vi "SimpleLiveAppPostProcessing.vi"() -> ()   [LabVIEW 2018]
uses:
  D:/SVN/PM/sdk/AppSamples/LabVIEWSamples/trunk/Release/2018/Dependencies/PVCamNET.dll
  Dependencies/PVCamNET.dll
panel:
  in  "Value":dbl
  in  "Post Processing":string(combo)
  in  "Exposure Time":dbl
  in  "Live":bool
  in  "Camera Status":bool
  in  "Uninit":bool
  in  "Live stop":bool
  in  "Live start":bool
  in  "Init":bool
  # "SimpleLiveAppPostProcessing.vi\n\nDescription:\nThis sample code lets the user use post processing\nfeature in an event driven structure.\n\nSteps to run:\n1. Click \"Run\"\n2. Click \"Open\"\n3. Enter Exposure Time\n4. Choose Post Processing feature\n5. Update Value\n6. Click \"Live start\"\n7. Click \"Live stop\"\n8. Click \"Close\""
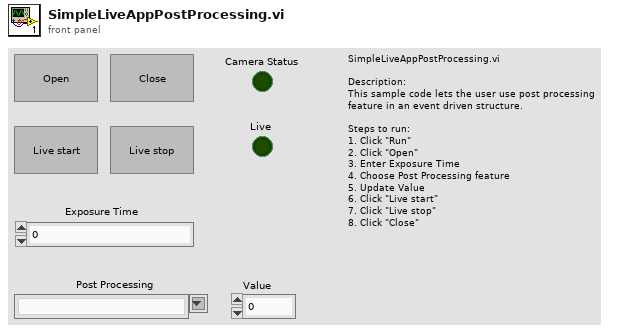
[diagram p1: front panel]
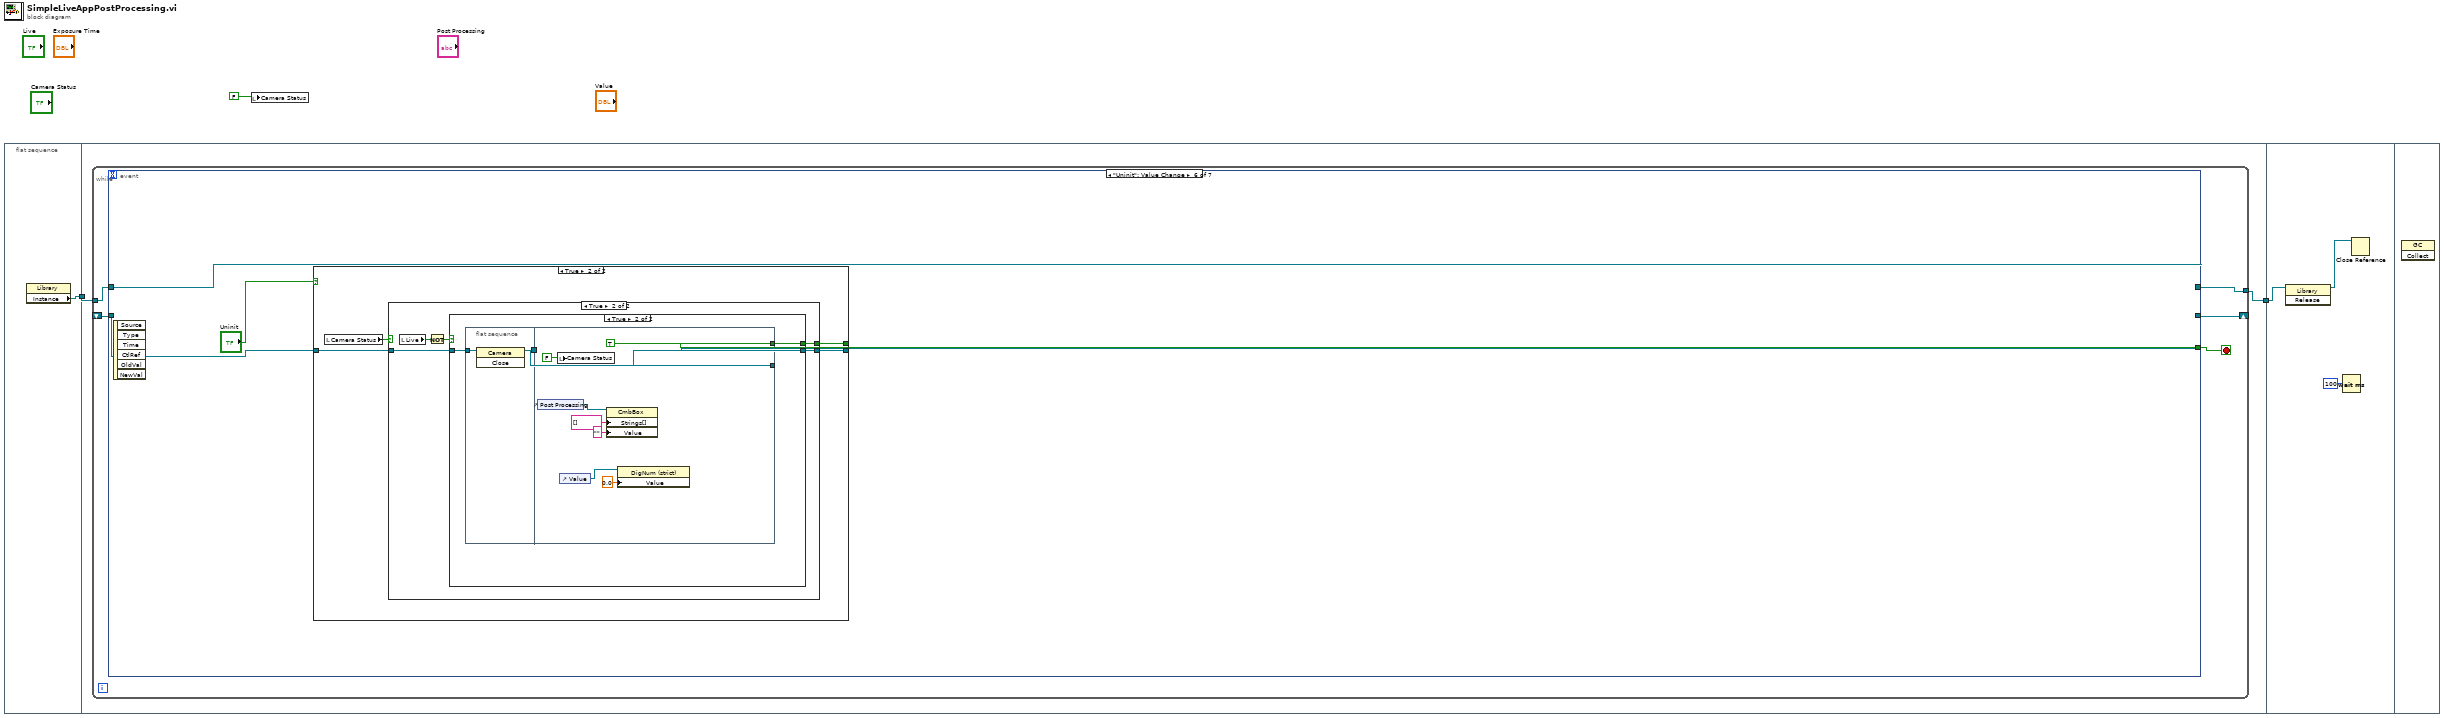
[diagram p0: block diagram]
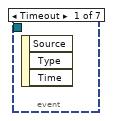
[diagram p2: hidden frame]
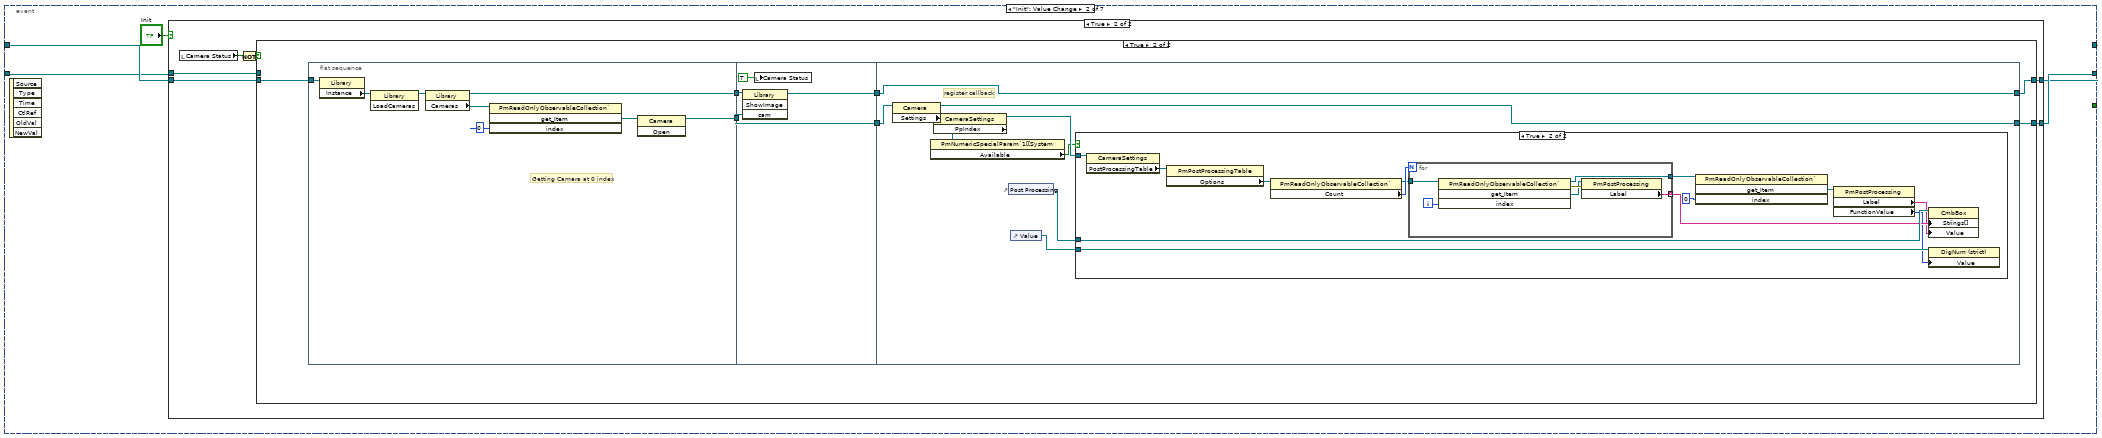
[diagram p3: hidden frame]
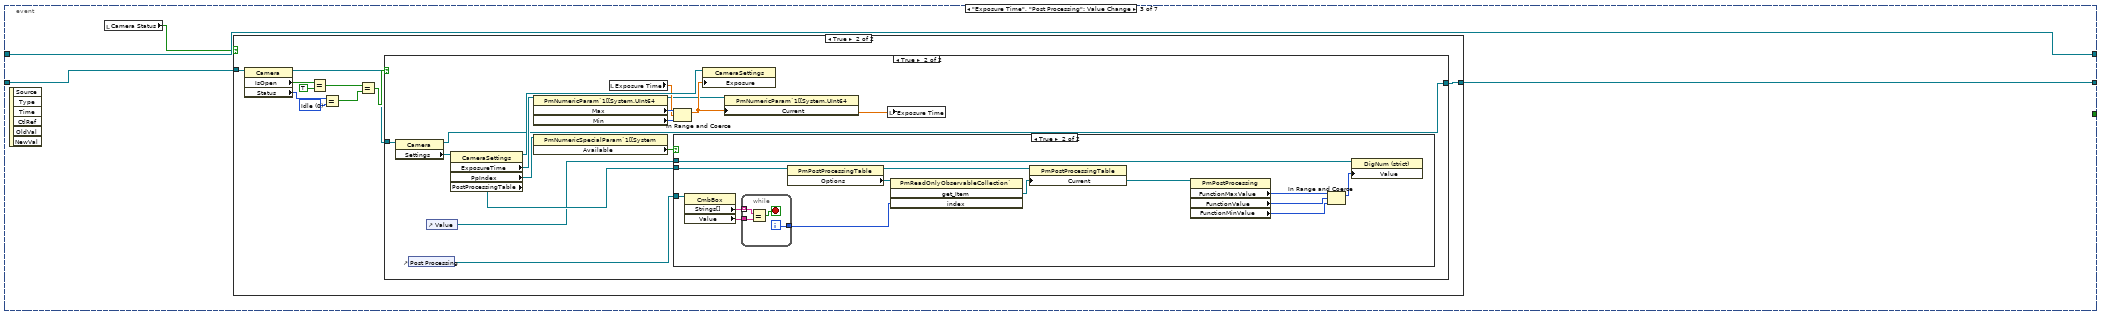
[diagram p7: hidden frame]
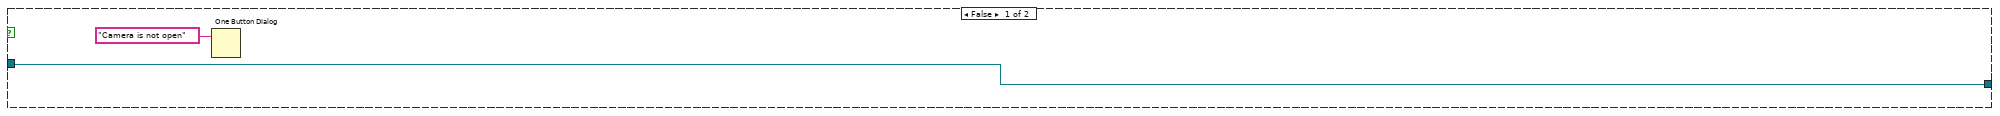
[diagram p8: hidden frame]
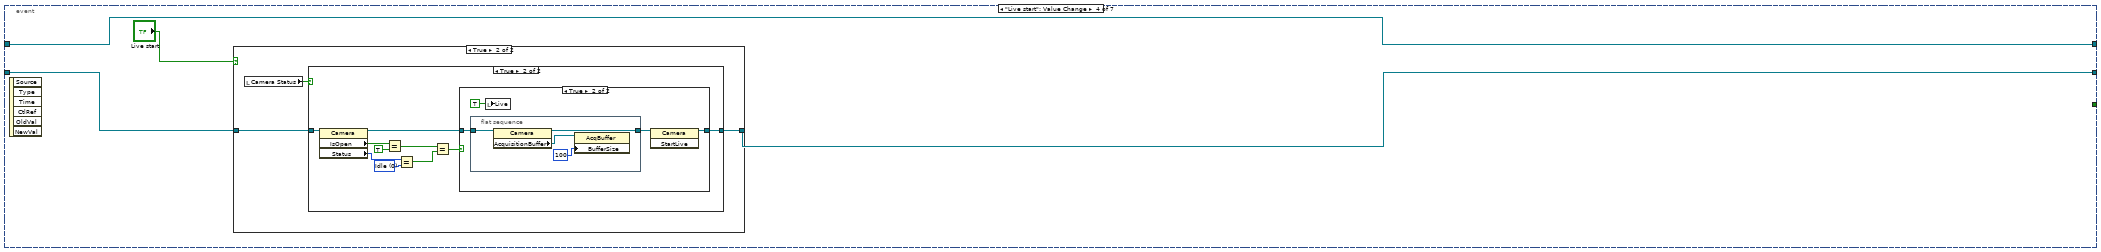
[diagram p11: hidden frame]
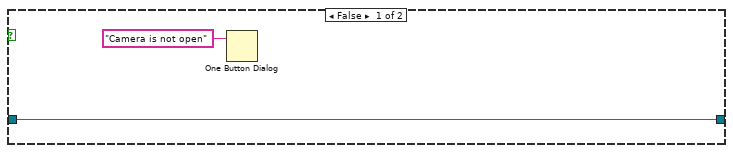
[diagram p13: hidden frame]
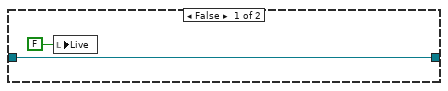
[diagram p14: hidden frame]
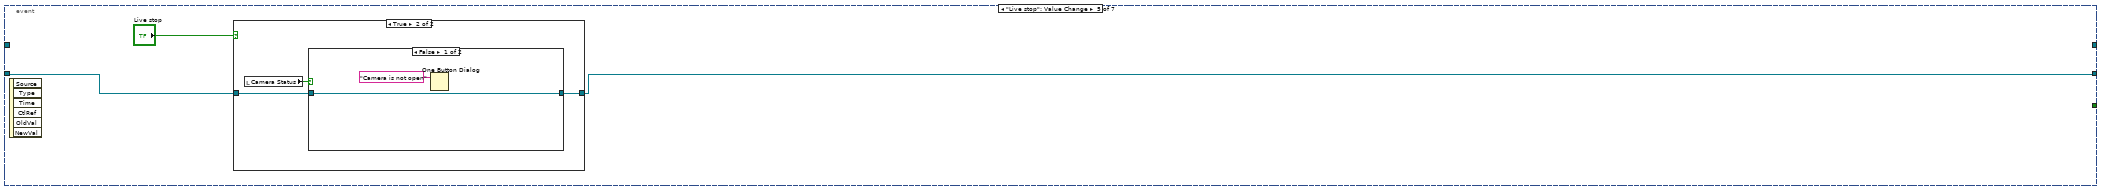
[diagram p15: hidden frame]
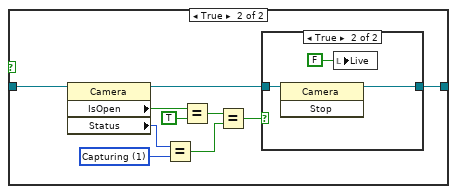
[diagram p17: hidden frame]
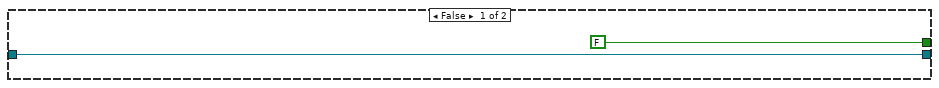
[diagram p19: hidden frame]
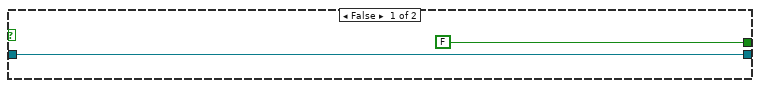
[diagram p20: hidden frame]
diagram:
  n1 = flat-sequence {
    tunnel: [w4] -> w3
    tunnel: w3 -> [w6]
    tunnel: [w5] -> w2
    tunnel: w2 -> [w243]
    frame #0 {
      n2 = property class="Library"() -> ("Instance"=w4:refnum<k24>)  [unwired: 2 in, 2 out]
    }
    frame #1 {
      n3 = while {
        tunnel: w6 -> [w11]
        shift-right: [w10] -> _
        shift-left: _ -> [w8]
        tunnel: [w9] -> w5
        stop <- w7 stop-if-true
        n4 = event shown="[5] \"Uninit\": Value Change" {
          selector: _ -> [_ _ _ _ _ _ _]
          dyn-events: _ -> [_ _ _ _ _ _ _]
          timeout: _ -> [_ _ _ _ _ _ _]
          tunnel: w11 -> [_ w16 w75 w123 _ w178 _]
          tunnel: [_ w15 w76 w124 w153 w179 w210] -> w10
          tunnel: [_ w14 w75 w123 _ w178 _] -> w9
          tunnel: w8 -> [_ w13 w77 w125 w154 w180 w212]
          tunnel: [_ _ _ _ _ w177 _] -> w7
          event Timeout {
            n5 = event-data() -> ()  [unwired: 1 in, 3 out]
          }
          event "Init": Value Change {
            n6 = event-data() -> ()  [unwired: 1 in, 6 out]
            n7 = case shown="True" "Init" {
              tunnel: w16 -> [w18 w24]
              tunnel: [w17 w23] -> w15
              tunnel: [w18 w22] -> w14
              tunnel: w13 -> [w17 w19]
              frame False {
              }
              frame True {
                n8 = local read "Camera Status"() -> (w21:bool)
                n9 = Not(x=w21) -> (.not. x?=w20:bool)
                n10 = case shown="True" w20 {
                  tunnel: w24 -> [w25 w31]
                  tunnel: [w26 w30] -> w23
                  tunnel: [w25 w29] -> w22
                  tunnel: w19 -> [w26 _]
                  frame False {
                  }
                  frame True {
                    n11 = flat-sequence {
                      tunnel: w31 -> [w37]
                      tunnel: [w38] -> w33
                      tunnel: [w34] -> w32
                      tunnel: w33 -> [w44]
                      tunnel: w32 -> [w45]
                      tunnel: [w45] -> w28
                      tunnel: [w43] -> w27
                      tunnel: [w54] -> w29
                      tunnel: [w46] -> w30
                      tunnel: w28 -> [w47]
                      tunnel: w27 -> [w54]
                      frame #0 {
                        # "Getting Camera at 0 index"
                        n12 = property class="Library"(reference=w37) -> ("Instance"=w36:refnum<k24>)  [unwired: 1 in, 2 out]
                        n13 = invoke class="Library" method="LoadCameras"(reference=w36) -> (reference out=w35:refnum<k24>)  [unwired: 2 in, 2 out]
                        n14 = property class="Library"(reference=w35) -> (reference out=w38:refnum<k24>, "Cameras"=w41:refnum<k24>)  [unwired: 1 in, 1 out]
                        n15 = invoke class="PmReadOnlyObservableCollection`" method="get_Item"(reference=w41, "index"=0) -> ("get_Item"=w39:refnum<k24>)  [unwired: 2 in, 3 out]
                        n16 = invoke class="Camera" method="Open"(reference=w39) -> (reference out=w34:refnum<k24>)  [unwired: 2 in, 2 out]
                      }
                      frame #1 {
                        n17 = invoke class="Library" method="ShowImage"(reference=w44, "cam"=w45) -> (reference out=w43:refnum<k24>)  [unwired: 2 in, 3 out]
                        n18 = local write "Camera Status"(TRUE ("Camera Status")) -> ()
                      }
                      frame #2 {
                        # "register callback"
                        n19 = property class="Camera"(reference=w47) -> (reference out=w46:refnum<k24>, "Settings"=w50:refnum<k24>)  [unwired: 1 in, 1 out]
                        n20 = property class="CameraSettings"(reference=w50) -> (reference out=w51:refnum<k24>, "PpIndex"=w49:refnum<k24>)  [unwired: 1 in, 1 out]
                        n21 = property class="PmNumericSpecialParam`1[[System"(reference=w49) -> ("Available"=w48:bool)  [unwired: 1 in, 2 out]
                        n22 = control-ref of="Post Processing"() -> (w52:refnum<vi>)
                        n23 = control-ref of="Value"() -> (w53:refnum<vi>)
                        n24 = case shown="True" w48 {
                          tunnel: w51 -> [_ w67]
                          tunnel: w52 -> [_ w59]
                          tunnel: w53 -> [_ w56]
                          frame False {
                          }
                          frame True {
                            n25 = property class="CameraSettings"(reference=w67) -> ("PostProcessingTable"=w66:refnum<k24>)  [unwired: 1 in, 2 out]
                            n26 = property class="PmPostProcessingTable"(reference=w66) -> ("Options"=w65:refnum<k24>)  [unwired: 1 in, 2 out]
                            n27 = property class="PmReadOnlyObservableCollection`"(reference=w65) -> (reference out=w63:refnum<k24>, "Count"=w64:i32)  [unwired: 1 in, 1 out]
                            n28 = for {
                              N: w64 -> [_]
                              tunnel: w63 -> [w73]
                              tunnel: [w69] -> w58 mode=indexing
                              tunnel: [w68] -> w62
                              i -> [w72]
                              n29 = invoke class="PmReadOnlyObservableCollection`" method="get_Item"(reference=w73, "index"=w72) -> (reference out=w68:refnum<k24>, error out=w71:errorcluster, "get_Item"=w70:refnum<k24>)  [unwired: 2 in, 1 out]
                              n30 = property class="PmPostProcessing"(reference=w70, error in=w71) -> ("Label"=w69:string)  [unwired: 2 out]
                            }
                            n31 = invoke class="PmReadOnlyObservableCollection`" method="get_Item"(reference=w62, "index"=0) -> ("get_Item"=w60:refnum<k24>)  [unwired: 2 in, 3 out]
                            n32 = property class="PmPostProcessing"(reference=w60) -> ("Label"=w57:string, "FunctionValue"=w55:i32)  [unwired: 1 in, 2 out]
                            n33 = property class="CmbBox"(reference=w59, "Strings[]"=w58, "Value"=w57) -> ()  [unwired: 1 in, 2 out]
                            n34 = property class="DigNum (strict)"(reference=w56, "Value"=w55) -> ()  [unwired: 1 in, 2 out]
                          }
                        }
                      }
                    }
                  }
                }
              }
            }
          }
          event "Exposure Time", "Post Processing": Value Change {
            n35 = event-data() -> ()  [unwired: 1 in, 6 out]
            n36 = local read "Camera Status"() -> (w74:bool)
            n37 = case shown="True" w74 {
              tunnel: w77 -> [w79 w83]
              tunnel: [w79 w80] -> w76
              frame False {
                n38 = One Button Dialog(message="Camera is not open") -> ()  [unwired: 1 in, 1 out]
              }
              frame True {
                w88 = 0 items=["Idle", "Capturing"] ("Status")
                n39 = property class="Camera"(reference=w83) -> (reference out=w81:refnum<k24>, "IsOpen"=w87:bool, "Status"=w89:i32)  [unwired: 1 in, 1 out]
                n40 = Equal?(x=w87, y=TRUE) -> (x = y?=w85:bool)
                n41 = Equal?(x=w89, y=w88) -> (x = y?=w84:bool)
                n42 = Equal?(x=w85, y=w84) -> (x = y?=w82:bool)
                n43 = case shown="True" w82 {
                  tunnel: w81 -> [w90 w105]
                  tunnel: [w90 w98] -> w80
                  frame False {
                  }
                  frame True {
                    n44 = property class="Camera"(reference=w105) -> (reference out=w98:refnum<k24>, "Settings"=w104:refnum<k24>)  [unwired: 1 in, 1 out]
                    n45 = control-ref of="Post Processing"() -> (w95:refnum<vi>)
                    n46 = control-ref of="Value"() -> (w93:refnum<vi>)
                    n47 = property class="CameraSettings"(reference=w104) -> (reference out=w100:refnum<k24>, "ExposureTime"=w101:refnum<k24>, "PpIndex"=w97:refnum<k24>, "PostProcessingTable"=w94:refnum<k24>)  [unwired: 1 in, 1 out]
                    n48 = property class="PmNumericParam`1[[System.UInt64"(reference=w101) -> (reference out=w91:refnum<k24>, "Max"=w103:u64, "Min"=w102:u64)  [unwired: 1 in, 1 out]
                    n49 = property class="PmNumericSpecialParam`1[[System"(reference=w97) -> ("Available"=w96:bool)  [unwired: 1 in, 2 out]
                    n50 = local read "Exposure Time"() -> (w99:dbl)
                    n51 = In Range and Coerce(upper limit=w103, x=w99, lower limit=w102) -> (coerced(x)=w92:dbl)  [unwired: 1 out]
                    n52 = case shown="True" w96 {
                      tunnel: w94 -> [_ w108]
                      tunnel: w95 -> [_ w116]
                      tunnel: w93 -> [_ w114]
                      frame False {
                      }
                      frame True {
                        n53 = property class="CmbBox"(reference=w116) -> ("Strings[]"=w118:string[], "Value"=w117:string)  [unwired: 1 in, 2 out]
                        n54 = while {
                          tunnel: w118 -> [w122] mode=indexing
                          tunnel: w117 -> [w121]
                          tunnel: [w119] -> w107
                          i -> [w119]
                          stop <- w120 stop-if-true
                          n55 = Equal?(x=w122, y=w121) -> (x = y?=w120:bool)
                        }
                        n56 = property class="PmPostProcessingTable"(reference=w108) -> (reference out=w106:refnum<k24>, "Options"=w115:refnum<k24>)  [unwired: 1 in, 1 out]
                        n57 = invoke class="PmReadOnlyObservableCollection`" method="get_Item"(reference=w115, "index"=w107) -> ("get_Item"=w109:refnum<k24>)  [unwired: 2 in, 3 out]
                        n58 = property class="PmPostProcessingTable"(reference=w106, "Current"=w109) -> ()  [unwired: 1 in, 2 out]
                        n59 = property class="PmPostProcessing"(reference=w109) -> ("FunctionMaxValue"=w112:i32, "FunctionValue"=w111:i32, "FunctionMinValue"=w110:i32)  [unwired: 1 in, 2 out]
                        n60 = In Range and Coerce(upper limit=w112, x=w111, lower limit=w110) -> (coerced(x)=w113:i32)  [unwired: 1 out]
                        n61 = property class="DigNum (strict)"(reference=w114, "Value"=w113) -> ()  [unwired: 1 in, 2 out]
                      }
                    }
                    n62 = property class="CameraSettings"(reference=w100, "Exposure"=w92) -> ()  [unwired: 1 in, 2 out]
                    n63 = property class="PmNumericParam`1[[System.UInt64"(reference=w91, "Current"=w92) -> ()  [unwired: 1 in, 2 out]
                    n64 = local write "Exposure Time"(w92) -> ()
                  }
                }
              }
            }
          }
          event "Live start": Value Change {
            n65 = event-data() -> ()  [unwired: 1 in, 6 out]
            n66 = case shown="True" "Live start" {
              tunnel: w125 -> [w127 w130]
              tunnel: [w127 w129] -> w124
              frame False {
              }
              frame True {
                n67 = local read "Camera Status"() -> (w128:bool)
                n68 = case shown="True" w128 {
                  tunnel: w130 -> [w131 w136]
                  tunnel: [w131 w134] -> w129
                  frame False {
                    n69 = One Button Dialog(message="Camera is not open") -> ()  [unwired: 1 in, 1 out]
                  }
                  frame True {
                    w141 = 0 items=["Idle", "Capturing"] ("Status")
                    n70 = property class="Camera"(reference=w136) -> (reference out=w135:refnum<k24>, "IsOpen"=w140:bool, "Status"=w142:i32)  [unwired: 1 in, 1 out]
                    n71 = Equal?(x=w140, y=TRUE) -> (x = y?=w138:bool)
                    n72 = Equal?(x=w142, y=w141) -> (x = y?=w137:bool)
                    n73 = Equal?(x=w138, y=w137) -> (x = y?=w133:bool)
                    n74 = case shown="True" w133 {
                      tunnel: w135 -> [w144 w146]
                      tunnel: [w144 w147] -> w134
                      frame False {
                        n75 = local write "Live"(FALSE ("Live 2")) -> ()
                      }
                      frame True {
                        n76 = flat-sequence {
                          tunnel: w146 -> [w152]
                          tunnel: [w149] -> w145
                          frame #0 {
                            n77 = property class="Camera"(reference=w152) -> (reference out=w149:refnum<k24>, "AcquisitionBuffer"=w151:refnum<k24>)  [unwired: 1 in, 1 out]
                            n78 = property class="AcqBuffer"(reference=w151, "BufferSize"=100) -> ()  [unwired: 1 in, 2 out]
                          }
                        }
                        n79 = local write "Live"(TRUE ("Live")) -> ()
                        n80 = invoke class="Camera" method="StartLive"(reference=w145) -> (reference out=w147:refnum<k24>)  [unwired: 2 in, 2 out]
                      }
                    }
                  }
                }
              }
            }
          }
          event "Live stop": Value Change {
            n81 = event-data() -> ()  [unwired: 1 in, 6 out]
            n82 = case shown="True" "Live stop" {
              tunnel: w154 -> [w156 w159]
              tunnel: [w156 w158] -> w153
              frame False {
              }
              frame True {
                n83 = local read "Camera Status"() -> (w157:bool)
                n84 = case shown="False" w157 {
                  tunnel: w159 -> [w161 w171]
                  tunnel: [w161 w168] -> w158
                  frame False {
                    n85 = One Button Dialog(message="Camera is not open") -> ()  [unwired: 1 in, 1 out]
                  }
                  frame True {
                    w166 = 1 items=["Idle", "Capturing"] ("Status")
                    n86 = property class="Camera"(reference=w171) -> (reference out=w169:refnum<k24>, "IsOpen"=w165:bool, "Status"=w167:i32)  [unwired: 1 in, 1 out]
                    n87 = Equal?(x=w167, y=w166) -> (x = y?=w162:bool)
                    n88 = Equal?(x=w165, y=TRUE) -> (x = y?=w163:bool)
                    n89 = Equal?(x=w163, y=w162) -> (x = y?=w170:bool)
                    n90 = case shown="True" w170 {
                      tunnel: w169 -> [w172 w175]
                      tunnel: [w172 w174] -> w168
                      frame False {
                      }
                      frame True {
                        n91 = invoke class="Camera" method="Stop"(reference=w175) -> (reference out=w174:refnum<k24>)  [unwired: 2 in, 2 out]
                        n92 = local write "Live"(FALSE ("Live 2")) -> ()
                      }
                    }
                  }
                }
              }
            }
          }
          event "Uninit": Value Change {
            n93 = event-data() -> ()  [unwired: 1 in, 6 out]
            n94 = case shown="True" "Uninit" {
              tunnel: w180 -> [w182 w186]
              tunnel: [w182 w185] -> w179
              tunnel: [FALSE ("Camera Status") w183] -> w177
              frame False {
              }
              frame True {
                n95 = local read "Camera Status"() -> (w184:bool)
                n96 = case shown="True" w184 {
                  tunnel: w186 -> [w188 w193]
                  tunnel: [w188 w192] -> w185
                  tunnel: [FALSE ("Camera Status") w191] -> w183
                  frame False {
                  }
                  frame True {
                    n97 = local read "Live"() -> (w189:bool)
                    n98 = Not(x=w189) -> (.not. x?=w190:bool)
                    n99 = case shown="True" w190 {
                      tunnel: w193 -> [w195 w198]
                      tunnel: [w195 w197] -> w192
                      tunnel: [FALSE ("Camera Status") w196] -> w191
                      frame False {
                      }
                      frame True {
                        n100 = flat-sequence {
                          tunnel: w198 -> [w201]
                          tunnel: [w200] -> w199
                          tunnel: [w209] -> w197
                          tunnel: w199 -> [w209]
                          tunnel: [TRUE ("Camera Status")] -> w196
                          frame #0 {
                            n101 = invoke class="Camera" method="Close"(reference=w201) -> (reference out=w200:refnum<k24>)  [unwired: 2 in, 2 out]
                          }
                          frame #1 {
                            n102 = control-ref of="Post Processing"() -> (w206:refnum<vi>)
                            n103 = local write "Camera Status"(FALSE ("Camera Status")) -> ()
                            n104 = control-ref of="Value"() -> (w203:refnum<vi>)
                            n105 = property class="CmbBox"(reference=w206, "Strings[]"=string[] [] ("Strings []"), "Value"="") -> ()  [unwired: 1 in, 2 out]
                            n106 = property class="DigNum (strict)"(reference=w203, "Value"=0.0) -> ()  [unwired: 1 in, 2 out]
                          }
                        }
                      }
                    }
                  }
                }
              }
            }
          }
          event "Value": Value Change {
            n107 = event-data() -> ()  [unwired: 1 in, 6 out]
            n108 = local read "Camera Status"() -> (w211:bool)
            n109 = case shown="True" w211 {
              tunnel: w212 -> [w213 w218]
              tunnel: [w213 w215] -> w210
              frame False {
                n110 = One Button Dialog(message="Camera is not open") -> ()  [unwired: 1 in, 1 out]
              }
              frame True {
                w223 = 0 items=["Idle", "Capturing"] ("Status")
                n111 = property class="Camera"(reference=w218) -> (reference out=w217:refnum<k24>, "IsOpen"=w222:bool, "Status"=w224:i32)  [unwired: 1 in, 1 out]
                n112 = Equal?(x=w222, y=TRUE) -> (x = y?=w220:bool)
                n113 = Equal?(x=w224, y=w223) -> (x = y?=w219:bool)
                n114 = Equal?(x=w220, y=w219) -> (x = y?=w216:bool)
                n115 = case shown="True" w216 {
                  tunnel: w217 -> [w225 w231]
                  tunnel: [w225 w226] -> w215
                  frame False {
                  }
                  frame True {
                    n116 = property class="Camera"(reference=w231) -> (reference out=w226:refnum<k24>, "Settings"=w230:refnum<k24>)  [unwired: 1 in, 1 out]
                    n117 = property class="CameraSettings" props=["PpIndex", "PpParam", "PostProcessingTable"](reference=w230) -> ("PpIndex"=w229:refnum<k24>, "PpParam"=w227:refnum<k24>)  [unwired: 1 in, 3 out]
                    n118 = property class="PmNumericSpecialParam`1[[System"(reference=w229) -> ("Available"=w228:bool)  [unwired: 1 in, 2 out]
                    n119 = case shown="True" w228 {
                      tunnel: w227 -> [_ w237]
                      frame False {
                      }
                      frame True {
                        # "1. Check if the input is in the right range\n2. Set the input value\n3. Display the set value"
                        n120 = control-ref of="Value"() -> (w241:refnum<vi>)
                        n121 = property class="PmPostProcessingParam"(reference=w237) -> (reference out=w232:refnum<k24>, "Max"=w240:u32, "Min"=w239:u32)  [unwired: 1 in, 1 out]
                        n122 = property class="DigNum (strict)"(reference=w241) -> (reference out=w235:refnum<vi>, "Value"=w236:dbl)  [unwired: 1 in, 1 out]
                        n123 = In Range and Coerce(upper limit=w240, x=w236, lower limit=w239) -> (coerced(x)=w233:dbl)  [unwired: 1 out]
                        n124 = property class="PmPostProcessingParam"(reference=w232, "Current"=w233) -> (reference out=w238:refnum<k24>)  [unwired: 1 in, 1 out]
                        n125 = property class="PmPostProcessingParam"(reference=w238) -> ("Current"=w234:u32)  [unwired: 1 in, 2 out]
                        n126 = property class="DigNum (strict)"(reference=w235, "Value"=w234) -> ()  [unwired: 1 in, 2 out]
                      }
                    }
                  }
                }
              }
            }
          }
        }
      }
    }
    frame #2 {
      n127 = invoke class="Library" method="Release"(reference=w243) -> (reference out=w244:refnum<k24>)  [unwired: 2 in, 2 out]
      n128 = Wait (ms)(milliseconds to wait=u32 100) -> ()  [unwired: 1 out]
      n129 = Close Reference(reference=w244) -> ()  [unwired: 1 in, 1 out]
    }
    frame #3 {
      n130 = invoke class="GC" method="Collect"() -> ()  [unwired: 3 in, 3 out]
    }
  }
  n131 = local write "Camera Status"(FALSE ("Camera Status")) -> ()
